vi "Wake-up Helper Loop for Pkt Loss Calc.vi"(8 "error in":errorcluster) -> (0 "error out":errorcluster)   [LabVIEW 2019, in "Acquisition.lvlib"]
doc: "Helper Loop for calculating packet loss for running 5 second average.\n_____\nCreated using DQMH Event Scripter 7.0.0.1280."
uses:
  Acquisition.lvlib
  Wake-up Helper Loop for Pkt Loss Calc Argument--cluster.ctl
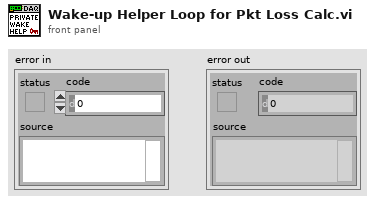
[diagram p1: front panel]
types:
  T1 = typedef "Acquisition.lvlib/Wake-up Helper Loop for Pkt Loss Calc Argument--cluster.ctl" = cluster{"Boolean":bool}
  T2 = typedef "Acquisition.lvlib/Request Events--cluster.ctl" = cluster{"Stop Module":refnum<user-event>, "Show Panel":refnum<user-event>, "Hide Panel":refnum<user-event>, "Get Module Execution Status":refnum<user-event>, "Show Diagram":refnum<user-event>, "Stop Acquiring":refnum<user-event>, "Wakeup Helper Loop":refnum<user-event>, "Change Settings":refnum<user-event>, "Calibrate DAQ":refnum<user-event>, "Start Acquiring":refnum<user-event>, "Command_TestData":refnum<user-event>, "Check WiFi AP":refnum<user-event>, "Command_NoiseData":refnum<user-event>, "Command_LiveData":refnum<user-event>, "Command_ImpedanceData":refnum<user-event>, "Command_GoToIdle":refnum<user-event>, "Soft Trigger":refnum<user-event>, "Start IMP Acquiring":refnum<user-event>, "Stop IMP acquiring":refnum<user-event>, "Start GND Loop acquiring":refnum<user-event>, "IMP data updated":refnum<user-event>, "Start CNV Acquiring":refnum<user-event>, "Start EOC Acquiring":refnum<user-event>, "Private":cluster{"Wake-up Helper Loop for Pkt Loss Calc":refnum<user-event>, "Stop Pkt Loss Calc":refnum<user-event>, "Update Packet ID":refnum<user-event>, "Calculate Packet Loss":refnum<user-event>}, "Command_GndImpedanceData":refnum<user-event>}
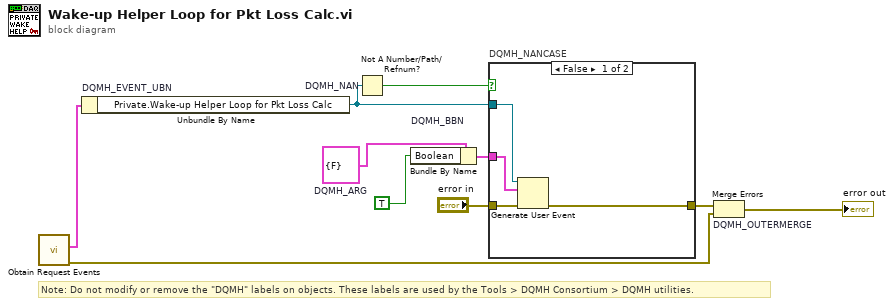
[diagram p0: block diagram]
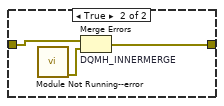
[diagram p2: hidden frame]
diagram:
  w4 = T1 {"Boolean"=FALSE}  # DQMH_ARG
  # "Note: Do not modify or remove the \"DQMH\" labels on objects. These labels are used by the Tools > DQMH Consortium > DQMH utilities."
  n1 = call "Obtain Request Events.vi"() -> ("error out"=w2:errorcluster, "Acquisition Request Events"=w1:T2)  [unwired: 10 in]
  n2 = Unbundle By Name "DQMH_EVENT_UBN"(w1) -> ("Private.Wake-up Helper Loop for Pkt Loss Calc"=w6:refnum<user-event>)
  n3 = Not A Number/Path/Refnum? "DQMH_NAN"(number/path/refnum=w6) -> (NaN/Path/Refnum?=w7:bool)
  n4 = Bundle By Name "DQMH_BBN"(cluster=w4, "Boolean"=TRUE) -> (w8:T1)
  n5 = case "DQMH_NANCASE" shown="False" w7 {
    tunnel: "error in" -> [w14 w17]
    tunnel: [w13 w16] -> w5
    tunnel: w6 -> [w12 _]
    tunnel: w8 -> [w11 _]
    frame False {
      n6 = Generate User Event(user event=w12, event data cluster=w11, error in=w14) -> (error out=w13:errorcluster)  [unwired: 1 in, 1 out]
    }
    frame True {
      n7 = call "Module Not Running--error.vi"() -> ("error out"=w15:errorcluster)  [unwired: 11 in]
      n8 = Merge Errors "DQMH_INNERMERGE"(w17, w15) -> (w16:errorcluster)
    }
  }
  n9 = Merge Errors "DQMH_OUTERMERGE"(w5, w2) -> (→"error out":errorcluster)
